vi "initialise.vi"(8 "error in (no error)":errorcluster, 11 "NetworkCamera in":refnum<class "NetworkCamera.lvclass">) -> (0 "error out":errorcluster, 3 "NetworkCamera out":refnum<class "NetworkCamera.lvclass">)   [LabVIEW 2009, in "Hardware.lvlib" / "HWControllers.lvlib" / "NetworkCamera.lvclass"]
uses:
  NetworkCamera.lvclass
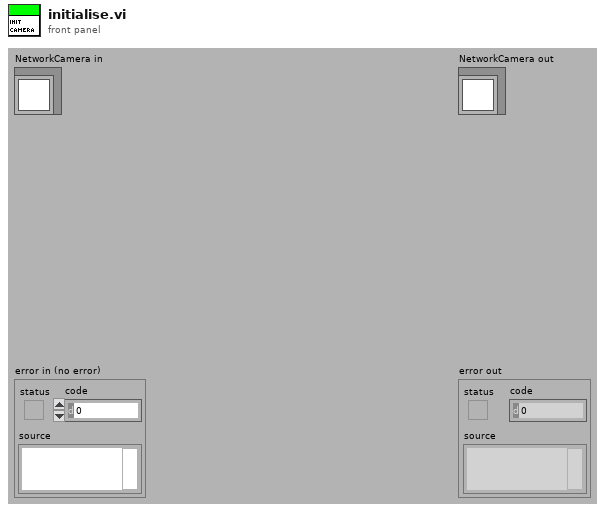
[diagram p1: front panel]
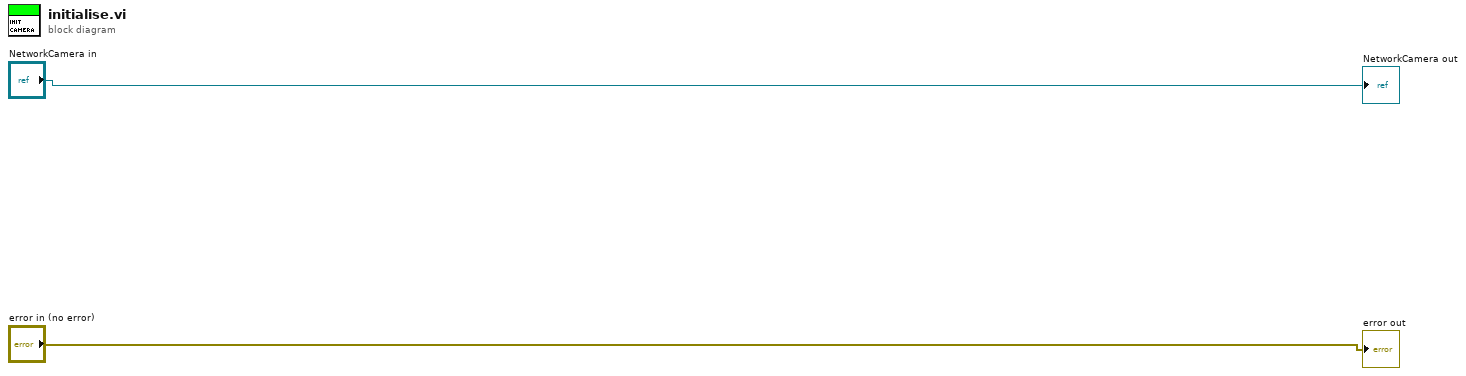
[diagram p0: block diagram]
diagram:
  "error out" <- "error in (no error)"
  "NetworkCamera out" <- "NetworkCamera in"
